vi "action_define.vi"(1 "action":T2, 2 "action data":T1[](array[typedef]) {"par 4" format="%.2f"; "par 3" format="%.2f"; "par 2" format="%.2f"; "par" format="%.2f"}, 3 "par":dbl format="%.2f", 4 "par 2":dbl format="%.2f", 5 "error in (no error)":errorcluster, 6 "idx":i32, 7 "par 3":dbl format="%.2f", 8 "idx 2":i32, 9 "par 4":dbl format="%.2f", 10 "no duplicate":bool, 11 "skip old":bool, 13 "force immidiate":bool) -> (16 "action data out":T1[](array[typedef]) {"par 4" format="%.2f"; "par 3" format="%.2f"; "par 2" format="%.2f"; "par" format="%.2f"}, 19 "error out":errorcluster)   [LabVIEW 2010, in "OSA.lvclass"]
doc: "Useful in parallell loops. \n\nCreate action data cluster which is placed in action queue by Thorlabs_FTS_LVXX_action_set.vi. Actions can be dequeued by Thorlabs_FTS_LVXX_action_get.vi and Thorlabs_FTS_LVXX_action_dequeue.vi in named order. See also Example Asynchronous acquisition.\n\nNote - do not call Thorlabs_FTS_LVXX_action_dequeue.vi until action is complete."
uses:
  OSA.lvclass
  typeDef/queue_action.ctl
  misc_examples/action_data.ctl
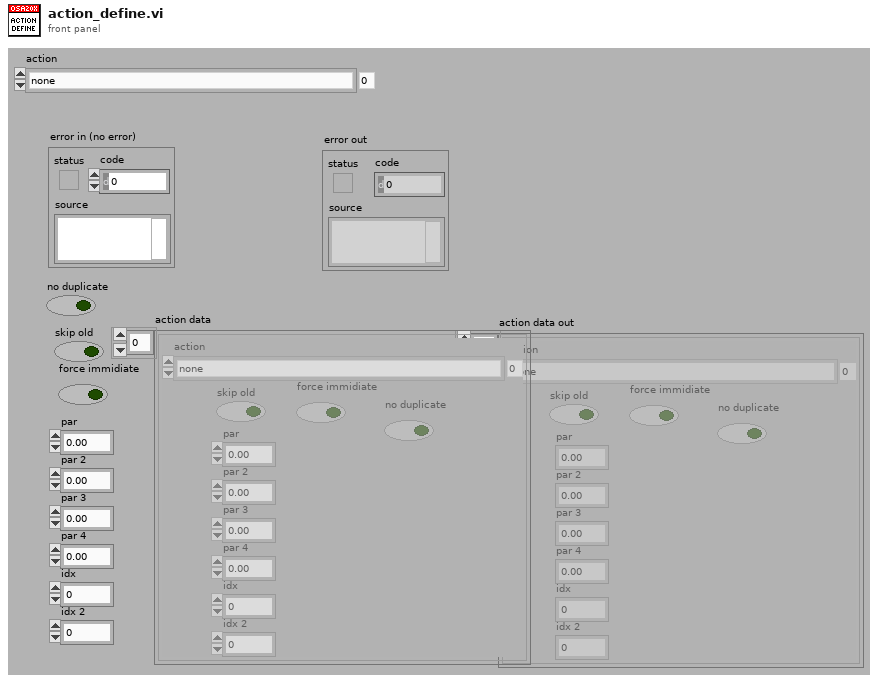
[diagram p1: front panel]
types:
  T1 = typedef "OSA.lvclass/action_data.ctl" = cluster{"action":T2, "skip old":bool, "force immidiate":bool, "par":dbl, "par 2":dbl, "par 3":dbl, "par 4":dbl, "idx":i32, "idx 2":i32, "no duplicate":bool}
  T2 = typedef "OSA.lvclass/queue_action.ctl" = enum16{"none", "stop", "GUI_plotInterferogram", "GUI_plotSpectrum", "GUI_plotInterferogramRescale", "GUI_plotSpectrumRescale", "GUI_plotInterferogramReset", "GUI_plotSpectrumReset", "GUI_plotInterferogramAutoScaleY", "GUI_plotSpectrumAutoScaleY", "GUI_plotInterferogramZoomOut", "GUI_plotSpectrumZoomOut", "GUI_plotInterferogramPane", "GUI_plotSpectrumPane", "GUI_plotInterferogramZoomMouse", "GUI_plotSpectrumZoomMouse", "ENVIRONMENT temperature", "ENVIRONMENT pressure", "MODE_resolution set", "MODE_resolution get", "MODE_sensitivity set", "MODE_sensitivity get", "MODE_PDTemperature set", "MODE_PDTemperature get", "REBOOT/RESET firmware", "ACQASYNC_acquireSingleSpectrum", "ACQASYNC_continuous start", "ACQASYNC_continuous stop\n", "ACQASYNC_get last interferogram", "ACQASYNC_get last spectrum", "ACQASYNC_get last waveNr", "ACQOPT_interferogram smoothing set", "ACQOPT_interferogram smoothing get", "ACQOPT_spectrum smoothing set", "ACQOPT_spectrum smoothing get", "ACQOPT_apodisation type set", "ACQOPT_apodisation type get", "ACQOPT_phase correction type set", "ACQOPT_phase correction type get", "ACQOPT_acqIntervall_set", "ACQOPT_acqIntervall_get", "ACQOPT_average spectrum set", "ACQOPT_average spectrum get", "ACQOPT_rolling average set", "ACQOPT_rolling average get", "ACQOPT_zero fill factor set", "ACQOPT_zero fill factor get", "ACQOPT_cycle counting set", "ACQOPT_cycle counting get", "ACQOPT_air measure option set", "ACQOPT_air measure option get", "ACQOPT_gainLevel auto get", "ACQOPT_gainLevel auto set", "ACQOPT_gainLevel get", "ACQOPT_gainLevel set", "ACQOPT_getAll", "INSTRUMENT_PROPERTY_range_WaveNr_min", "INSTRUMENT_PROPERTY_range_WaveNr_max", "INSTRUMENT_PROPERTY_reference_wavelength_cm^-1", "INSTRUMENT_PROPERTY_samplesPerRefPeriod", "INSTRUMENT_PROPERTY_resolution_waveNrPercm", "INSTRUMENT_PROPERTY_availableGainLevels", "INSTRUMENT_PROPERTY_status", "CONVERT", "ANALYSE_POWER", "ANALYSE_PEAKS", "ANALYSE_WAVELENGTH", "ANALYSE_SPECTRUM", "ANALYSE_INTERFEROGRAM", "ANALYSE_COHERENCE_LENGTH", "MATH", "MATH_power", "MATH_peaks", "FILE", "miscellaneous"}
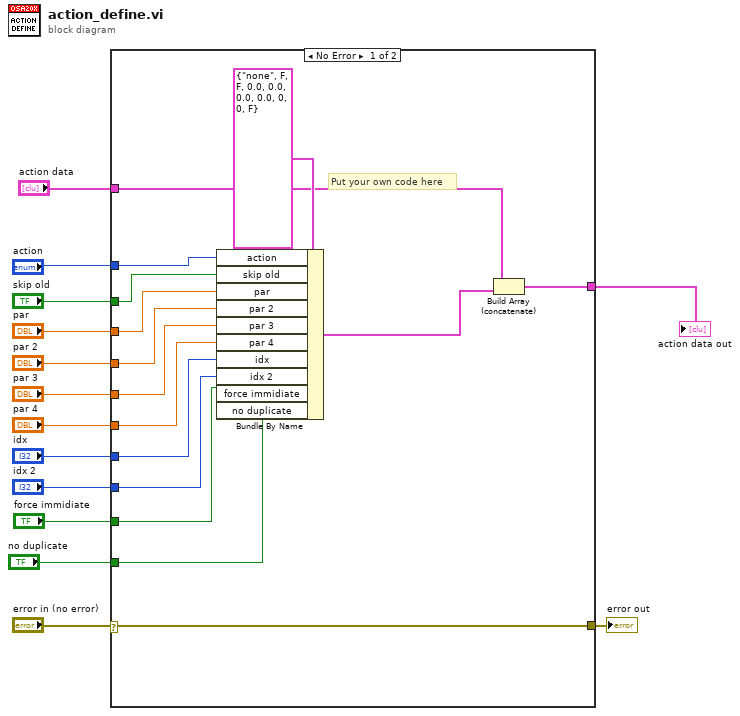
[diagram p0: block diagram]
diagram:
  n1 = case shown="No Error" "error in (no error)" {
    selector: "error in (no error)" -> [w29 w31]
    tunnel: [w29 w31] -> w14
    tunnel: "action" -> [w27 _]
    tunnel: "skip old" -> [w26 _]
    tunnel: "par" -> [w25 _]
    tunnel: "par 2" -> [w24 _]
    tunnel: "par 3" -> [w23 _]
    tunnel: "par 4" -> [w22 _]
    tunnel: "idx" -> [w21 _]
    tunnel: "idx 2" -> [w20 _]
    tunnel: "action data" -> [w19 w30]
    tunnel: [w17 w30] -> w3
    tunnel: "force immidiate" -> [w16 _]
    tunnel: "no duplicate" -> [w15 _]
    frame No Error {
      # "Put your own code here"
      n2 = Bundle By Name(cluster=T1 {"action"=enum."none", "skip old"=FALSE, "force immidiate"=FALSE, "par"=0.0, "par 2"=0.0, "par 3"=0.0, "par 4"=0.0, "idx"=0, "idx 2"=0, "no duplicate"=FALSE} ("element"), "action"=w27, "skip old"=w26, "par"=w25, "par 2"=w24, "par 3"=w23, "par 4"=w22, "idx"=w21, "idx 2"=w20, "force immidiate"=w16, "no duplicate"=w15) -> (w18:T1)
      n3 = Build Array (concatenate)(w19, w18) -> (w17:T1[])
    }
    frame Error {
      # "Error"
    }
  }
  "error out" <- w14
  "action data out" <- w3
